vi "GPOutApp.vi"() -> ()   [LabVIEW 2010]
panel:
  in  "Boolean":bool
  in  "stop":bool
  in  "ICImagingControl":refnum<k7>(container)
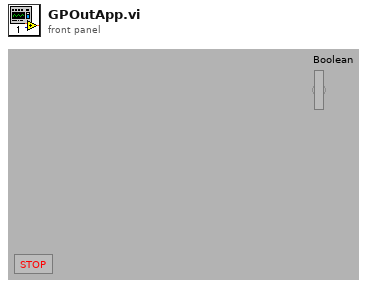
[diagram p1: front panel]
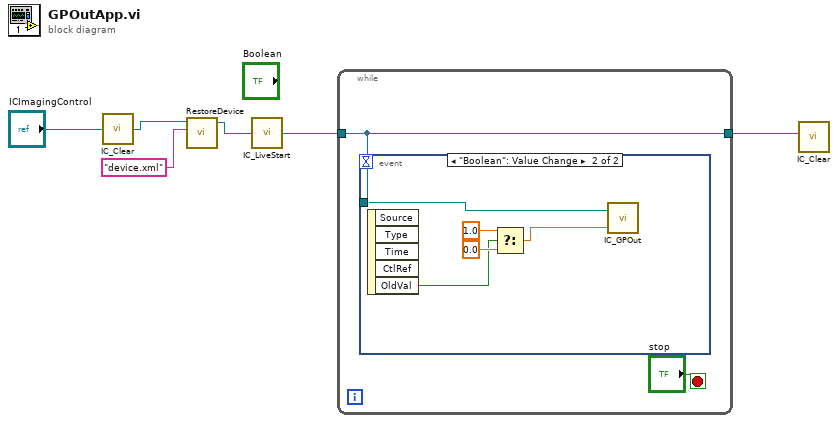
[diagram p0: block diagram]
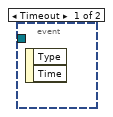
[diagram p2: hidden frame]
diagram:
  n1 = call <userlib>:"IC_Clear.vi"("ICImagingControl 2"="ICImagingControl") -> ("ICImagingControl"=w3:refnum<k7>)
  n2 = call <userlib>:"RestoreDevice.vi"("Filename"="device.xml", "ICImagingControl"=w3) -> ("ICImagingControl 2"=w2:refnum<k7>)  [unwired: 2 in, 2 out]
  n3 = call <userlib>:"IC_LiveStart.vi"("ICImagingControl 3"=w2) -> ("ICImagingControl 2"=w5:refnum<k7>)
  n4 = while {
    tunnel: w5 -> [w7]
    tunnel: [w7] -> w4
    stop <- "stop" stop-if-true
    n5 = event shown="[1] \"Boolean\": Value Change" {
      selector: _ -> [_ _]
      dyn-events: _ -> [_ _]
      timeout: _ -> [_ _]
      tunnel: w7 -> [_ w13]
      event Timeout {
        n6 = event-data() -> ()  [unwired: 1 in, 2 out]
      }
      event "Boolean": Value Change {
        n7 = event-data() -> ("OldVal"=w9:bool)  [unwired: 1 in, 4 out]
        n8 = Select(t=1.0, s=w9, f=0.0) -> (s? t:f=w12:dbl)
        n9 = call "IC_GPOut.vi"("GPOut Value"=w12, "ICImagingControl 3"=w13) -> ()  [unwired: 1 out]
      }
    }
  }
  n10 = call <userlib>:"IC_Clear.vi"("ICImagingControl 2"=w4) -> ()  [unwired: 1 out]
